vi "Atto DRY Interface Connect.vi"(8 "error in (no error)":errorcluster, 11 "COMPort":string) -> (0 "error out":errorcluster, 2 "function return":i32, 3 "COMPort out":string)   [LabVIEW 2016, in "attoDRYLib.lvlib"]
doc: "int32_t __cdecl AttoDRY_Interface_Connect(char COMPort[]);"
uses:
  <userlib>/attoDRYLib/attoDRYLib.lvlib
  <userlib>/attoDRYLib/attoDRYLib.dll
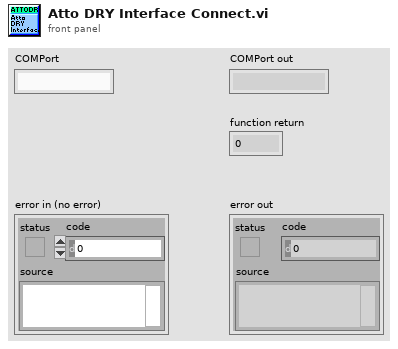
[diagram p1: front panel]
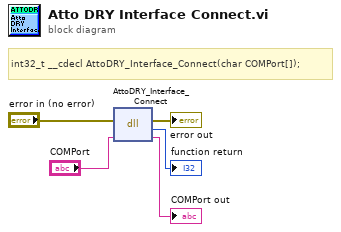
[diagram p0: block diagram]
diagram:
  # "int32_t __cdecl AttoDRY_Interface_Connect(char COMPort[]);"
  n1 = dll-call lib="C:/Program Files (x86)/National Instruments/LabVIEW 2016/user.lib/attoDRYLib/attoDRYLib.*" fn="AttoDRY_Interface_Connect"(error in="error in (no error)", "COMPort"="COMPort") -> (error out=→"error out":errorcluster, →"function return":i32, "COMPort"=→"COMPort out":string)  [unwired: 2 in, 1 out]
